vi "Generate Message with Arguments.vi"(11 "XML String":string) -> (3 "Message with Arguments":string)   [LabVIEW 2015, in "NI_Azure_Core.lvlib"]
uses:
  NI_Azure_Core.lvlib
  XML Parsing/NI_Azure_XML Parsing.lvlib
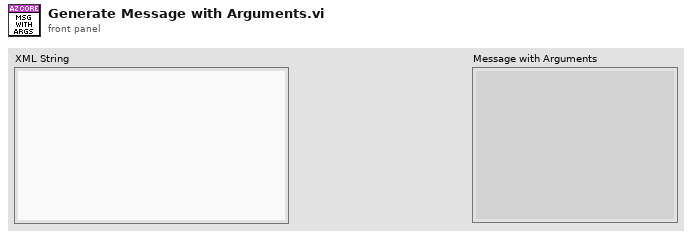
[diagram p1: front panel]
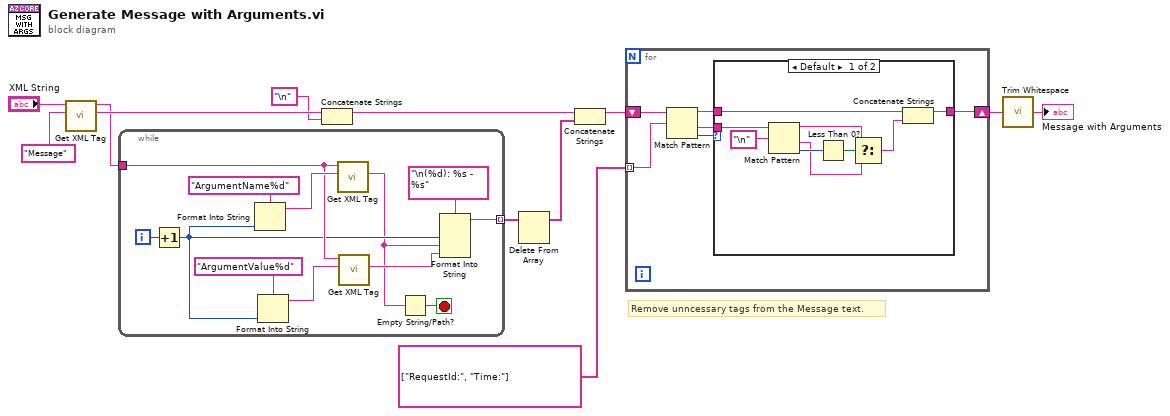
[diagram p0: block diagram]
diagram:
  # "Remove unncessary tags from the Message text."
  n1 = call "Get XML Tag.vi"("Tag name"="Message", "XML String in"="XML String") -> ("Tag value"=w12:string, "XML String dup"=w9:string)  [unwired: 5 in, 3 out]
  n2 = while {
    tunnel: w9 -> [w19]
    tunnel: [w15] -> w8 mode=indexing
    i -> [w24]
    stop <- w13 stop-if-true
    n3 = Increment(x=w24) -> (x+1=w17:i32)
    n4 = Format Into String(format string="ArgumentName%d", w17) -> (resulting string=w22:string)  [unwired: 2 in, 1 out]
    n5 = Format Into String(format string="ArgumentValue%d", w17) -> (resulting string=w20:string)  [unwired: 2 in, 1 out]
    n6 = call "Get XML Tag.vi"("Tag name"=w22, "XML String in"=w19) -> ("Tag value"=w14:string)  [unwired: 5 in, 4 out]
    n7 = call "Get XML Tag.vi"("Tag name"=w20, "XML String in"=w19) -> ("Tag value"=w16:string)  [unwired: 5 in, 4 out]
    n8 = Empty String/Path?(string/path=w14) -> (empty?=w13:bool)
    n9 = Format Into String(format string="\n(%d): %s - %s", w17, w14, w16) -> (resulting string=w15:string)  [unwired: 2 in, 1 out]
  }
  n10 = Concatenate Strings(w12, "\n" ("regular expression")) -> (w3:string)
  n11 = Delete From Array(array=w8) -> (array with subset deleted=w7:string[])  [unwired: 2 in, 1 out]
  n12 = Concatenate Strings(w3, w7) -> (w6:string)
  n13 = for {
    shift-right: [w26] -> w5
    shift-left: w6 -> [w30]
    tunnel: string[] ["RequestId:", "Time:"] -> [w29] mode=indexing
    n14 = Match Pattern(string=w30, regular expression=w29) -> (before substring=w27:string, after substring=w25:string, offset past match=w28:i32)  [unwired: 1 in, 1 out]
    n15 = case shown="Default" w28 {
      tunnel: w27 -> [w33 w40]
      tunnel: [w31 w40] -> w26
      tunnel: w25 -> [w39 _]
      frame Default {
        n16 = Match Pattern(string=w39, regular expression="\n") -> (before substring=w35:string, after substring=w34:string, offset past match=w37:i32)  [unwired: 1 in, 1 out]
        n17 = Less Than 0?(x=w37) -> (x < 0?=w36:bool)
        n18 = Select(t=w35, s=w36, f=w34) -> (s? t:f=w32:string)
        n19 = Concatenate Strings(w33, w32) -> (w31:string)
      }
      frame -1 {
      }
    }
  }
  n20 = call <vilib>:"Trim Whitespace.vi"("string"=w5) -> ("trimmed string"=→"Message with Arguments":string)  [unwired: 1 in]
